vi "Min.vi"(6 "Search Lines":T2[](array[typedef]) {"Edge Info"."Distance (Real-World)" format="%.2f"; "Edge Info"."Location (Real-World)"."Y" format="%.2g"; "Edge Info"."Location (Real-World)"."X" format="%.2f"; "Edge Info"."Noise" format="%.2f"; "Edge Info"."Location (Pixel)"."Y" format="%.2g"; "Edge Info"."Location (Pixel)"."X" format="%.2f"; "Edge Info"."Strength" format="%.2f"; "Edge Info"."Distance (Pixel)" format="%.2f"}, 9 "Last Edges":T1[](array[typedef]) {"Distance (Real-World)" format="%.2f"; "Location (Real-World)"."Y" format="%.2g"; "Location (Real-World)"."X" format="%.2f"; "Noise" format="%.2f"; "Location (Pixel)"."Y" format="%.2g"; "Location (Pixel)"."X" format="%.2f"; "Strength" format="%.2f"; "Distance (Pixel)" format="%.2f"}, 10 "First Edges":T1[](array[typedef]) {"Distance (Real-World)" format="%.2f"; "Location (Real-World)"."Y" format="%.2g"; "Location (Real-World)"."X" format="%.2f"; "Noise" format="%.2f"; "Location (Pixel)"."Y" format="%.2g"; "Location (Pixel)"."X" format="%.2f"; "Strength" format="%.2f"; "Distance (Pixel)" format="%.2f"}, 11 "Refnum in":T3) -> (2 "Array":cluster{"X":sgl, "Y":sgl}[](array[cluster]), 3 "Numeric":sgl)   [LabVIEW 2015]
uses:
  <vilib>/vision/Image Controls.llb/IMAQ Image.ctl
  <vilib>/vision/Measure.llb/Search Line.ctl
  <vilib>/vision/Measure.llb/Edge New.ctl
  <vilib>/vision/NI_Vision_Development_Module.lvlib
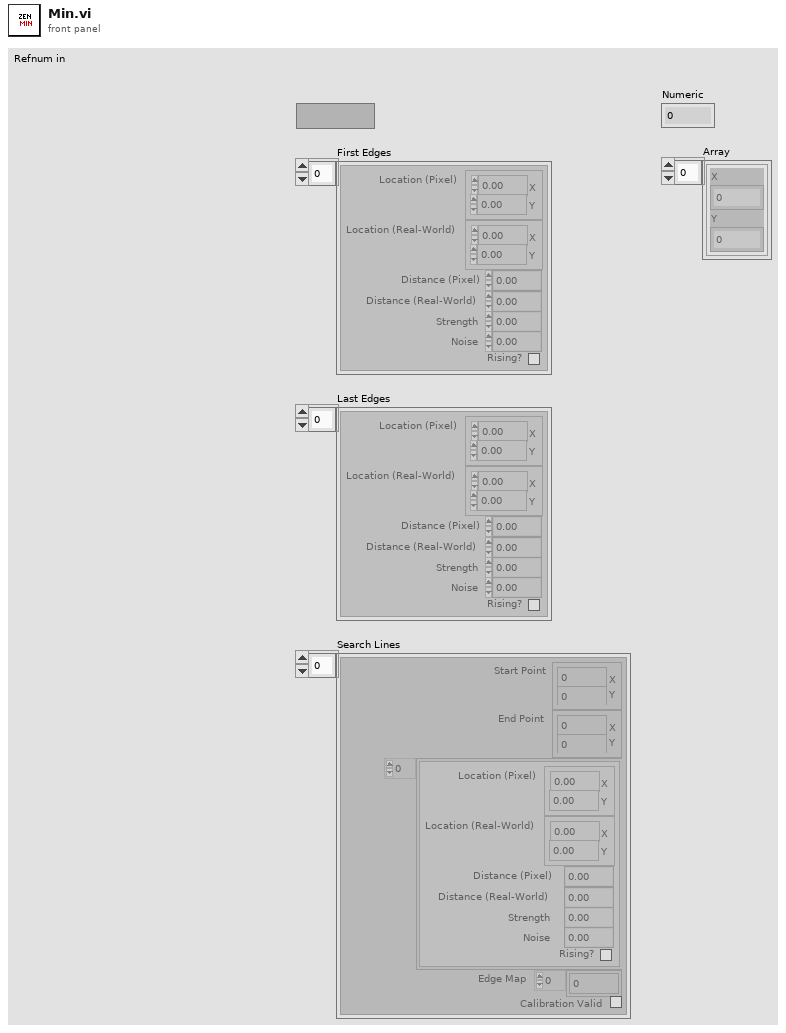
[diagram p1: front panel]
types:
  T1 = typedef "Edge New.ctl" = cluster{"Location (Pixel)":cluster{"X":sgl, "Y":sgl}, "Location (Real-World)":cluster{"X":sgl, "Y":sgl}, "Distance (Pixel)":dbl, "Distance (Real-World)":dbl, "Strength":dbl, "Noise":dbl, "Rising?":bool}
  T2 = typedef "Search Line.ctl" = cluster{"Start Point":cluster{"X":sgl, "Y":sgl}, "End Point":cluster{"X":sgl, "Y":sgl}, "Edge Info":T1[], "Edge Map":dbl[], "Calibration Valid":bool}
  T3 = typedef "IMAQ Image.ctl" = refnum<image>
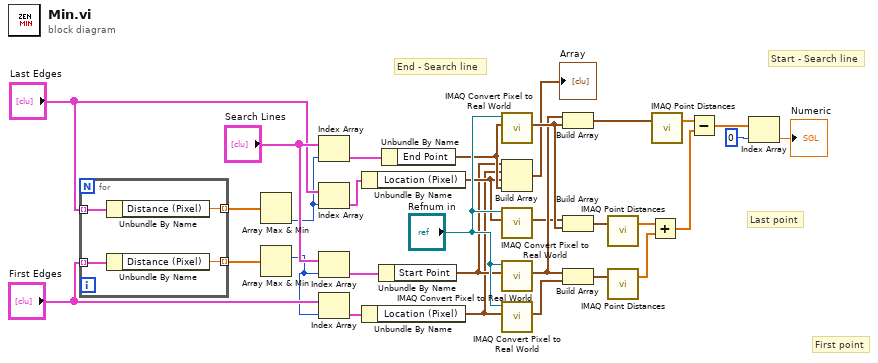
[diagram p0: block diagram]
diagram:
  # "Last point"
  # "First point"
  # "End - Search line"
  # "Start - Search line"
  n1 = for {
    tunnel: "First Edges" -> [w35] mode=indexing
    tunnel: [w34] -> w8 mode=indexing
    tunnel: "Last Edges" -> [w33] mode=indexing
    tunnel: [w32] -> w10 mode=indexing
    n2 = Unbundle By Name(w33) -> ("Distance (Pixel)"=w32:dbl)
    n3 = Unbundle By Name(w35) -> ("Distance (Pixel)"=w34:dbl)
  }
  n4 = Array Max & Min(array=w10) -> (min index (indices)=w2:i32)  [unwired: 3 out]
  n5 = Array Max & Min(array=w8) -> (max index (indices)=w1:i32)  [unwired: 3 out]
  n6 = Index Array(array="Search Lines", index=w2) -> (element=w12:T2)
  n7 = Index Array(array="Last Edges", index=w2) -> (element=w4:T1)
  n8 = Index Array(array="Search Lines", index=w1) -> (element=w5:T2)
  n9 = Index Array(array="First Edges", index=w1) -> (element=w3:T1)
  n10 = Unbundle By Name(w4) -> ("Location (Pixel)"=w17:cluster{"X":sgl, "Y":sgl})
  n11 = Unbundle By Name(w3) -> ("Location (Pixel)"=w13:cluster{"X":sgl, "Y":sgl})
  n12 = Unbundle By Name(w5) -> ("Start Point"=w14:cluster{"X":sgl, "Y":sgl})
  n13 = Unbundle By Name(w12) -> ("End Point"=w18:cluster{"X":sgl, "Y":sgl})
  n14 = call "IMAQ Convert Pixel to Real World"("Pixel Coordinates"=w18, "Calibrated Image"="Refnum in") -> ("Real World Coordinates"=w27:cluster{"X":sgl, "Y":sgl})  [unwired: 4 in, 5 out]
  n15 = Build Array(w14, w13, w17, w18) -> (→"Array":cluster{"X":sgl, "Y":sgl}[])
  n16 = call "IMAQ Convert Pixel to Real World"("Pixel Coordinates"=w17, "Calibrated Image"="Refnum in") -> ("Real World Coordinates"=w20:cluster{"X":sgl, "Y":sgl})  [unwired: 4 in, 5 out]
  n17 = call "IMAQ Convert Pixel to Real World"("Pixel Coordinates"=w14, "Calibrated Image"="Refnum in") -> ("Real World Coordinates"=w26:cluster{"X":sgl, "Y":sgl})  [unwired: 4 in, 5 out]
  n18 = call "IMAQ Convert Pixel to Real World"("Pixel Coordinates"=w13, "Calibrated Image"="Refnum in") -> ("Real World Coordinates"=w15:cluster{"X":sgl, "Y":sgl})  [unwired: 4 in, 5 out]
  n19 = Build Array(w26, w27) -> (w28:cluster{"X":sgl, "Y":sgl}[])
  n20 = Build Array(w20, w27) -> (w21:cluster{"X":sgl, "Y":sgl}[])
  n21 = Build Array(w26, w15) -> (w16:cluster{"X":sgl, "Y":sgl}[])
  n22 = call "IMAQ Point Distances"("Points"=w21) -> ("Distances"=w22:sgl[])  [unwired: 4 in, 1 out]
  n23 = call "IMAQ Point Distances"("Points"=w16) -> ("Distances"=w23:sgl[])  [unwired: 4 in, 1 out]
  n24 = Add(x=w22, y=w23) -> (x+y=w24:sgl[])
  n25 = call "IMAQ Point Distances"("Points"=w28) -> ("Distances"=w29:sgl[])  [unwired: 4 in, 1 out]
  n26 = Subtract(x=w29, y=w24) -> (x-y=w25:sgl[])
  n27 = Index Array(array=w25, index=0) -> (element=→"Numeric":sgl)
